vi "Read Description.vi"(11 "Decaf in":refnum<class "Decaf.lvclass">) -> (2 "Description":string)   [LabVIEW 2013, in "Decaf.lvclass"]
uses:
  Decaf.lvclass
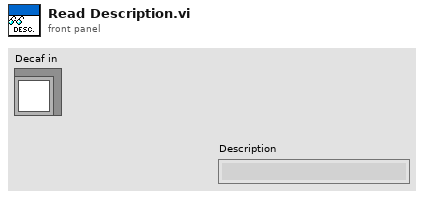
[diagram p1: front panel]
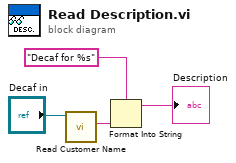
[diagram p0: block diagram]
diagram:
  n1 = call-dynamic "Read Customer Name.vi"("Beverage in"="Decaf in") -> ("Customer Name"=w1:string)  [unwired: 10 in]
  n2 = Format Into String(format string="Decaf for %s" ("Description"), w1) -> (resulting string=→"Description":string)  [unwired: 2 in, 1 out]
